vi "GetControlRef.vi"(0 "Controls[] In":refnum<vi>[](array[refnum]), 7 "Control Path":string[](array[string]), 11 "error In":errorcluster) -> (8 "Ctl Refnum":refnum<vi>, 15 "error out":errorcluster)   [LabVIEW 2016]
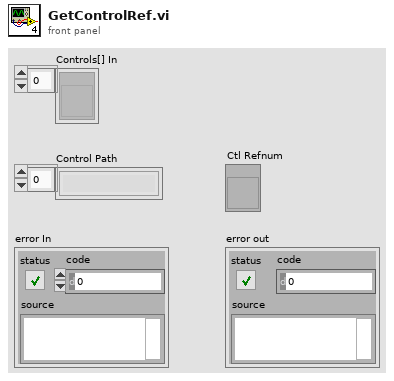
[diagram p1: front panel]
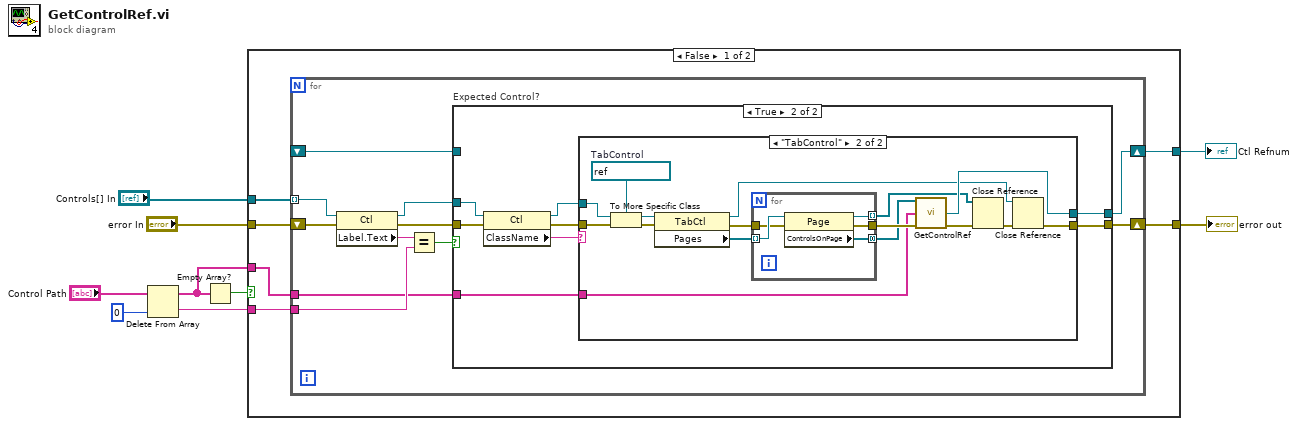
[diagram p0: block diagram]
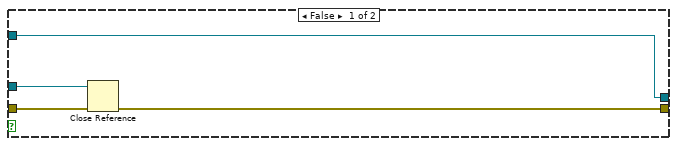
[diagram p2: hidden frame]
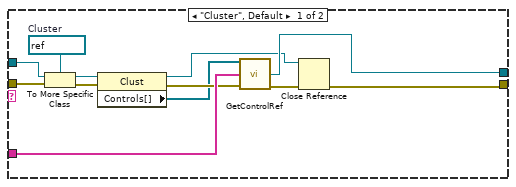
[diagram p3: hidden frame]
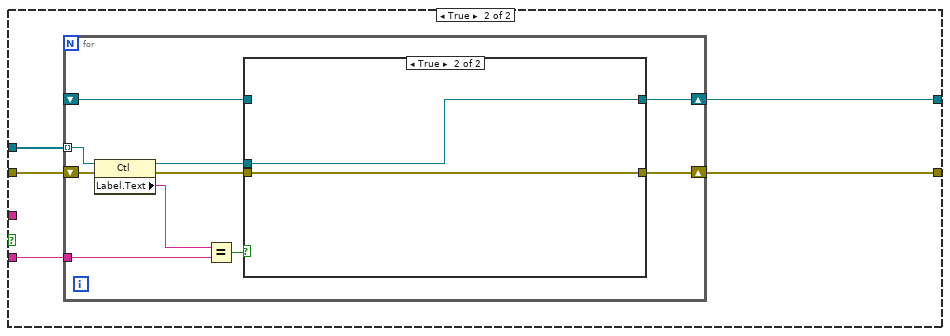
[diagram p4: hidden frame]
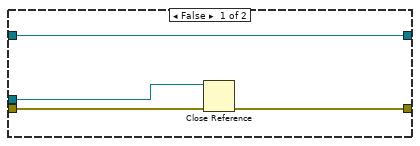
[diagram p5: hidden frame]
diagram:
  n1 = Delete From Array(array="Control Path", index=0) -> (deleted portion=w7:string, array with subset deleted=w3:string[])  [unwired: 1 in]
  n2 = Empty Array?(array=w3) -> (empty?=w8:bool)
  n3 = case shown="False" w8 {
    tunnel: "Controls[] In" -> [w15 w76]
    tunnel: w7 -> [w11 w75]
    tunnel: [w10 w74] -> w6
    tunnel: "error In" -> [w14 w73]
    tunnel: [w13 w72] -> w4
    tunnel: w3 -> [w12 _]
    frame False {
      n4 = for {
        tunnel: w15 -> [w24] mode=indexing
        tunnel: w12 -> [w19]
        tunnel: w11 -> [w22]
        shift-right: [w26] -> w13
        shift-left: w14 -> [w18]
        shift-right: [w17] -> w10
        shift-left: _ -> [w16]
        n5 = property class="Ctl"(reference=w24, error in=w18) -> (reference out=w21:refnum<vi>, error out=w23:errorcluster, "Label.Text"=w25:string)
        n6 = Equal?(x=w25, y=w22) -> (x = y?=w20:bool)
        n7 = case "Expected Control?" shown="True" w20 {
          tunnel: [w28 w32] -> w26
          tunnel: w23 -> [w30 w38]
          tunnel: w21 -> [w27 w36]
          tunnel: w19 -> [_ w33]
          tunnel: [w29 w31] -> w17
          tunnel: w16 -> [w29 _]
          frame False {
            n8 = Close Reference(reference=w27, error in (no error)=w30) -> (error out=w28:errorcluster)
          }
          frame True {
            n9 = property class="Ctl"(reference=w36, error in=w38) -> (reference out=w35:refnum<vi>, error out=w37:errorcluster, "ClassName"=w34:string)
            n10 = case shown="\"TabControl\"" w34 {
              tunnel: w37 -> [w48 w66]
              tunnel: w35 -> [w47 w65]
              tunnel: w33 -> [w45 w58]
              tunnel: [w41 w55] -> w32
              tunnel: [w42 w54] -> w31
              frame "Cluster", Default {
                w46 = refnum<vi> refnum  # Cluster
                n11 = To More Specific Class(target class=w46, reference=w47, error in=w48) -> (specific class reference=w50:refnum<vi>, error out=w49:errorcluster)
                n12 = property class="Clust"(reference=w50, error in=w49) -> (reference out=w40:refnum<vi>, error out=w44:errorcluster, "Controls[]"=w39:refnum<vi>[])
                n13 = call "GetControlRef.vi"("Controls[] In"=w39, "Control Path"=w45, "error In"=w44) -> ("Ctl Refnum"=w42:refnum<vi>, "error out"=w43:errorcluster)  [unwired: 11 in]
                n14 = Close Reference(reference=w40, error in (no error)=w43) -> (error out=w41:errorcluster)
              }
              frame "TabControl" {
                w64 = refnum<vi> refnum  # TabControl
                n15 = To More Specific Class(target class=w64, reference=w65, error in=w66) -> (specific class reference=w63:refnum<vi>, error out=w62:errorcluster)
                n16 = property class="TabCtl"(reference=w63, error in=w62) -> (reference out=w52:refnum<vi>, error out=w60:errorcluster, "Pages"=w61:refnum<vi>[])
                n17 = for {
                  tunnel: w61 -> [w71] mode=indexing
                  tunnel: w60 -> [w70]
                  tunnel: [w69] -> w59
                  tunnel: [w67] -> w51 mode=concatenating
                  tunnel: [w68] -> w53 mode=indexing
                  n18 = property class="Page"(reference=w71, error in=w70) -> (reference out=w68:refnum<vi>, error out=w69:errorcluster, "ControlsOnPage"=w67:refnum<vi>[])
                }
                n19 = call "GetControlRef.vi"("Controls[] In"=w51, "Control Path"=w58, "error In"=w59) -> ("Ctl Refnum"=w54:refnum<vi>, "error out"=w57:errorcluster)  [unwired: 11 in]
                n20 = Close Reference(reference=w53, error in (no error)=w57) -> (error out=w56:errorcluster)
                n21 = Close Reference(reference=w52, error in (no error)=w56) -> (error out=w55:errorcluster)
              }
            }
          }
        }
      }
    }
    frame True {
      n22 = for {
        tunnel: w76 -> [w86] mode=indexing
        tunnel: w75 -> [w84]
        shift-right: [w79] -> w72
        shift-left: w73 -> [w78]
        shift-right: [w81] -> w74
        shift-left: _ -> [w77]
        n23 = property class="Ctl"(reference=w86, error in=w78) -> (reference out=w82:refnum<vi>, error out=w80:errorcluster, "Label.Text"=w85:string)
        n24 = Equal?(x=w85, y=w84) -> (x = y?=w83:bool)
        n25 = case shown="True" w83 {
          tunnel: w82 -> [w87 w92]
          tunnel: [w89 w92] -> w81
          tunnel: w80 -> [w90 w91]
          tunnel: [w88 w91] -> w79
          tunnel: w77 -> [w89 _]
          frame False {
            n26 = Close Reference(reference=w87, error in (no error)=w90) -> (error out=w88:errorcluster)
          }
          frame True {
          }
        }
      }
    }
  }
  "Ctl Refnum" <- w6
  "error out" <- w4
